vi "SLSCAddPropertiesToSysDef.vi"(6 "Channel":T1={"Type"=enum."Input", "Units"="", "Default Value"=0.0, "Faultable"=TRUE, "Scalable"=TRUE}, 8 "error in (no error)":errorcluster, 10 "properties":T4[](array[typedef]), 11 "Section Ptr":T3 format="%.0x") -> (0 "error out":errorcluster)   [LabVIEW 2019]
uses:
  SLSC EDS API/JSON parsing/property.ctl
  <vilib>/NI VeriStand/Custom Device API/Custom Device Item Ref.ctl
  <vilib>/NI VeriStand/Custom Device API/Custom Device Channel.ctl
  <vilib>/NI VeriStand/Custom Device API/Custom Device Channel Type.ctl
  Shared/Constants.vi
  <vilib>/NI VeriStand/Custom Device API/Set Item Property (String).vi
  Shared/SLSC EDS Shared.lvlib
  <vilib>/NI VeriStand/Custom Device API/Custom Device API.lvlib
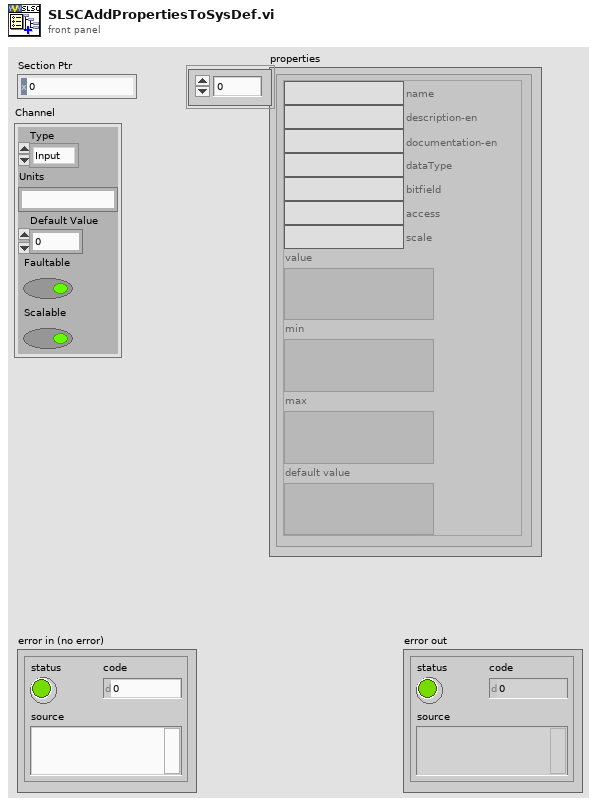
[diagram p1: front panel]
types:
  T1 = typedef "Custom Device API.lvlib/Custom Device Channel.ctl" = cluster{"Type":T2, "Units":string, "Default Value":dbl, "Faultable":bool, "Scalable":bool}
  T2 = typedef "Custom Device API.lvlib/Custom Device Channel Type.ctl" = enum16{"Input", "Output"}
  T3 = typedef "Custom Device API.lvlib/Custom Device Item Ref.ctl" = u64
  T4 = typedef "property.ctl" = cluster{"name":string, "description-en":string, "documentation-en":string, "dataType":string, "bitfield":string, "access":string, "scale":string, "value":variant, "min":variant, "max":variant, "default value":variant}
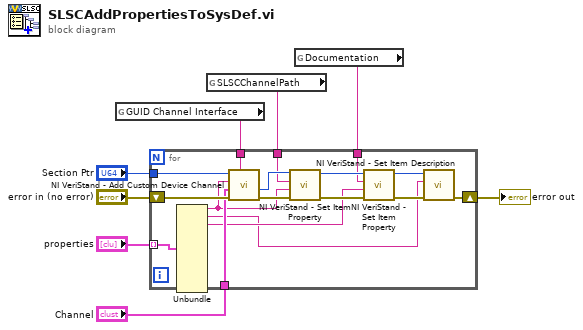
[diagram p0: block diagram]
diagram:
  n1 = global read "Constants.vi" "GUID Channel Interface"() -> (w7:string)
  n2 = global read "Constants.vi" "SLSCChannelPath"() -> (w6:string)
  n3 = global read "Constants.vi" "Documentation"() -> (w8:string)
  n4 = for {
    tunnel: "Section Ptr" -> [w21]
    shift-right: [w18] -> w3
    shift-left: "error in (no error)" -> [w20]
    tunnel: w6 -> [w23]
    tunnel: w7 -> [w22]
    tunnel: "properties" -> [w17] mode=indexing
    tunnel: "Channel" -> [w19]
    tunnel: w8 -> [w11]
    n5 = Unbundle(w17) -> ("name"=w16:string, "description-en"=w9:string, "documentation-en"=w10:string)  [unwired: 8 out]
    n6 = call <vilib>:"NI VeriStand - Add Custom Device Channel.vi"("GUID (Default Channel)"=w22, "error in (no error)"=w20, "Channel"=w19, "Channel Name"=w16, "Parent Ref in"=w21) -> ("error out"=w24:errorcluster, "Channel Ref"=w25:T3)  [unwired: 3 in, 2 out]
    n7 = call-poly <vilib>:"NI VeriStand - Set Item Property.vi"("error in (no error)"=w24, "Value"=w16, "Property Name"=w23, "Item Ref in"=w25) -> ("error out"=w14:errorcluster, "Item Ref out"=w15:T3)  [unwired: 5 in, 1 out]
    n8 = call-poly <vilib>:"NI VeriStand - Set Item Property.vi"("error in (no error)"=w14, "Value"=w10, "Property Name"=w11, "Item Ref in"=w15) -> ("error out"=w13:errorcluster, "Item Ref out"=w12:T3)  [unwired: 5 in, 1 out]
    n9 = call <vilib>:"NI VeriStand - Set Item Description.vi"("error in (no error)"=w13, "Description"=w9, "Item Ref in"=w12) -> ("error out"=w18:errorcluster)  [unwired: 6 in, 2 out]
  }
  "error out" <- w3
